vi "InsertDataToDB.vi"(7 "data":T1={"SN1"="01", "SN2"="02", "Test_Time"="03", "Test_Model"="04", "Test_Result"="05"}, 8 "error in (no error)":errorcluster, 10 "table":string="Table_1", 11 "DSN":string="Test_Report_1") -> (0 "error out":errorcluster, 2 "table?":bool=TRUE, 3 "error?":bool=TRUE)   [LabVIEW 2011]
uses:
  <vilib>/addons/database/Auxilliary.llb/DB Tools DataTypes.ctl
  <vilib>/addons/database/Connection.llb/DB Tools Open Connec (String).vi
  <vilib>/addons/database/NI_Database_API.lvlib
panel:
  out "column information":T3(array[cluster])=[{"name"="SN1", "database data type"=enum."String", "defined size"=50}, {"name"="SN2", "database data type"=enum."String", "defined size"=50}, {"name"="Test_Time", "database data type"=enum."String", "defined size"=50}, {"name"="Test_Model", "database data type"=enum."String", "defined size"=50}, {"name"="Test_Result", "database data type"=enum."String", "defined size"=50}]
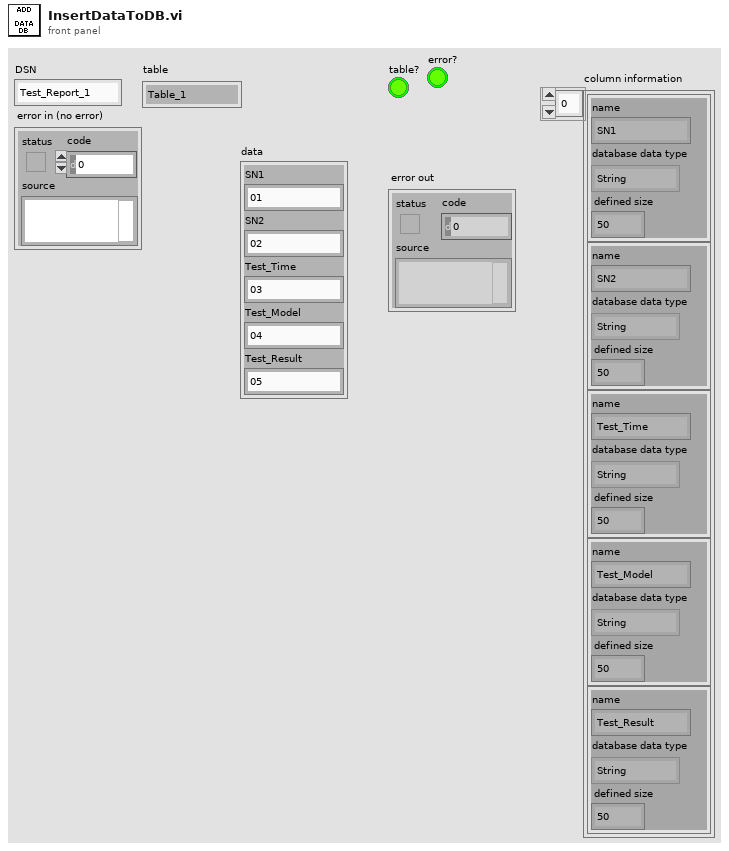
[diagram p1: front panel]
types:
  T1 = cluster{"SN1":string, "SN2":string, "Test_Time":string, "Test_Model":string, "Test_Result":string}
  T2 = typedef "NI_Database_API.lvlib/DB Tools DataTypes.ctl" = enum16{"String", "Long (I32)", "Single (SGL)", "Double (DBL)", "Date/Time", "Binary"}
  T3 = cluster{"name":string, "database data type":T2, "defined size":i32}[]
  T4 = typedef "NI_Database_API.lvlib/Conn ObjectReference.ctl" = refnum<k1>
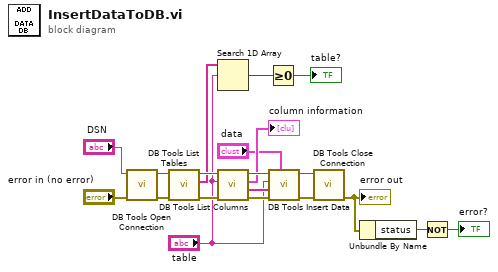
[diagram p0: block diagram]
diagram:
  n1 = call-poly <vilib>:"DB Tools Open Connection.vi"("error in (no error)"="error in (no error)", "connection information"="DSN") -> ("error out"=w18:errorcluster, "connection reference"=w19:T4)  [unwired: 6 in]
  n2 = call <vilib>:"DB Tools List Tables.vi"("error in (no error)"=w18, "connection reference"=w19) -> ("error out"=w16:errorcluster, "tables"=w8:string[], "connection reference out"=w17:T4)  [unwired: 3 in]
  n3 = Search 1D Array(1D array=w8, element="table") -> (index of element=w6:i32)  [unwired: 1 in]
  n4 = call <vilib>:"DB Tools List Columns.vi"("error in (no error)"=w16, "table"="table", "connection reference"=w17) -> ("error out"=w15:errorcluster, "columns"=w11:string[], "column information"=→"column information":T3, "connection reference out"=w13:T4)  [unwired: 1 in]
  n5 = Greater Or Equal To 0?(x=w6) -> (x >= 0?=→"table?":bool)
  n6 = call <vilib>:"DB Tools Insert Data.vi"("data"="data", "error in (no error)"=w15, "columns"=w11, "table"="table", "connection reference"=w13) -> ("error out"=w14:errorcluster, "connection reference out"=w12:T4)  [unwired: 5 in]
  n7 = call <vilib>:"DB Tools Close Connection.vi"("error in (no error)"=w14, "connection reference"=w12) -> ("error out"=w4:errorcluster)  [unwired: 5 in]
  "error out" <- w4
  n8 = Unbundle By Name(w4) -> ("status"=w3:bool)
  n9 = Not(x=w3) -> (.not. x?=→"error?":bool)
